vi "InitDir.vi"(8 "error in":errorcluster, 11 "DataIn":variant) -> (0 "error out":errorcluster, 3 "MainFGV_data":T1={"TestDir"=path "", "TestName"="", "Simulation"=FALSE, "task"="", "data_file"=refnum, "burts_file"=refnum, "log_file"=refnum, "Rate"=0.0, "SamplesPerChannel"=0.0, "AcqQueue"=refnum, "StartTime"=timestamp(0 s since 1904-01-01), "config_channels"=[], "DAQmx Device"="", "delta_burst"=15.0})   [LabVIEW 2016]
uses:
  MainFGV_data.ctl
  Settings/config_board.ctl
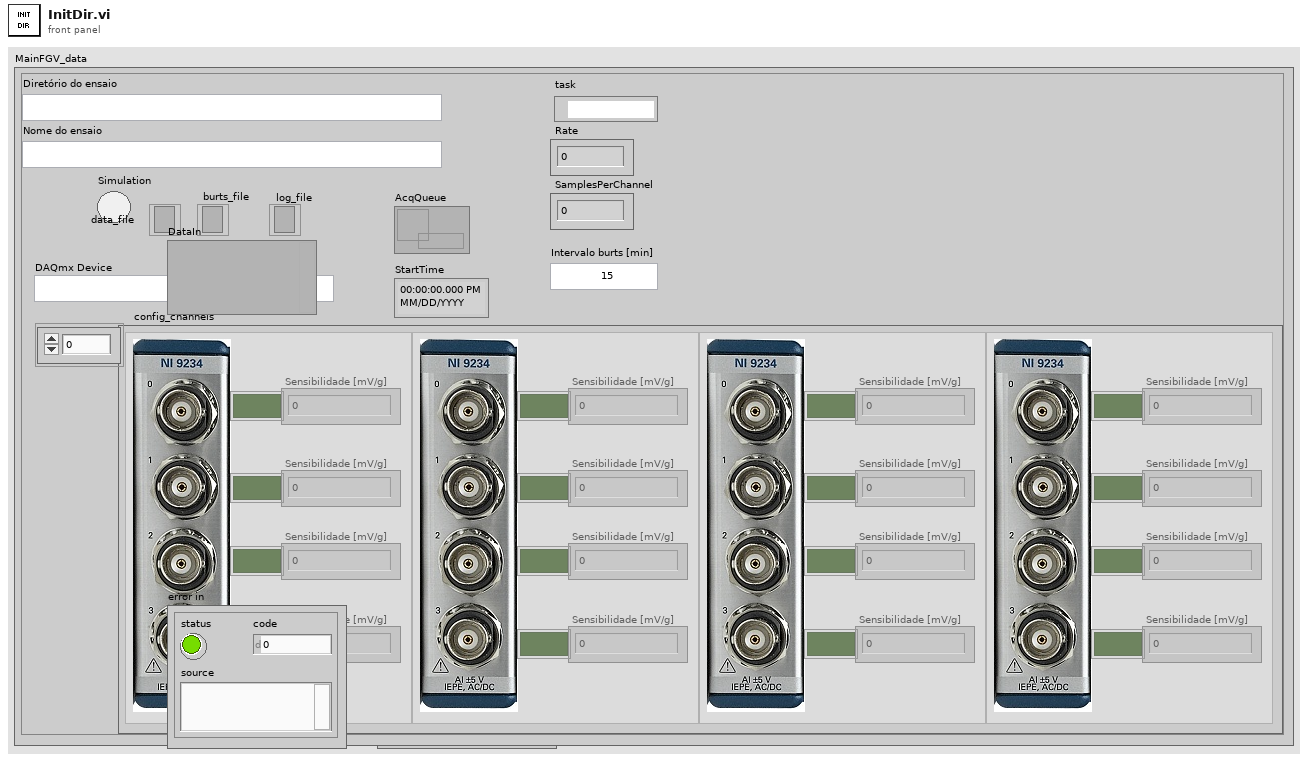
[diagram p1: front panel]
types:
  T1 = typedef "MainFGV_data.ctl" = cluster{"TestDir":path, "TestName":string, "Simulation":bool, "task":refnum<k21>, "data_file":refnum<file>, "burts_file":refnum<file>, "log_file":refnum<file>, "Rate":dbl, "SamplesPerChannel":dbl, "AcqQueue":refnum<queue>, "StartTime":timestamp, "config_channels":T2[], "DAQmx Device":tag, "delta_burst":dbl}
  T2 = typedef "config_board.ctl" = cluster{"Sens0":dbl, "Active0":bool, "Sens1":dbl, "Active1":bool, "Sens2":dbl, "Active2":bool, "Sens3":dbl, "Active3":bool}
  T3 = cluster{"simulation":bool, "TesrtDir":path, "TestName":string}
  T4 = enum16{"open", "replace", "create", "open or create", "replace or create", "replace or create with confirmation"}
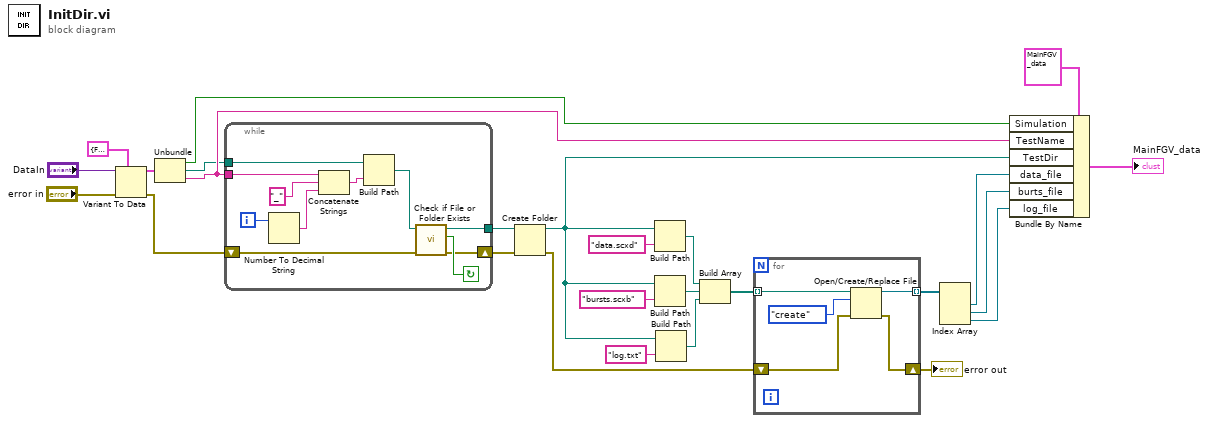
[diagram p0: block diagram]
diagram:
  n1 = Variant To Data(error in="error in", type=T3 {"simulation"=FALSE, "TesrtDir"=path "", "TestName"=""} ("output cluster"), Variant="DataIn") -> (data=w18:T3, error out=w20:errorcluster)
  n2 = Unbundle(w18) -> ("simulation"=w24:bool, "TesrtDir"=w22:path, "TestName"=w23:string)
  n3 = while {
    tunnel: w23 -> [w36]
    tunnel: w22 -> [w34]
    shift-right: [w30] -> w26
    shift-left: w20 -> [w32]
    tunnel: [w29] -> w25
    i -> [w37]
    stop <- w31 continue-if-true
    n4 = Number To Decimal String(number=w37) -> (decimal integer string=w28:string)  [unwired: 1 in]
    n5 = Concatenate Strings(w36, "_" ("string"), w28) -> (w35:string)
    n6 = Build Path(base path=w34, name or relative path=w35) -> (appended path=w33:path)
    n7 = call <vilib>:"Check if File or Folder Exists.vi"("error in (no error)"=w32, "path"=w33) -> ("error out"=w30:errorcluster, "file or folder exists?"=w31:bool, "dup path"=w29:path)  [unwired: 7 in]
  }
  n8 = Create Folder(path (use dialog)=w25, error in=w26) -> (created path=w11:path, error out=w6:errorcluster)  [unwired: 1 in, 1 out]
  n9 = Build Path(base path=w11, name or relative path="data.scxd") -> (appended path=w9:path)
  n10 = Build Path(base path=w11, name or relative path="bursts.scxb") -> (appended path=w10:path)
  n11 = Build Path(base path=w11, name or relative path="log.txt") -> (appended path=w8:path)
  n12 = Build Array(w9, w10, w8) -> (w7:path[])
  n13 = for {
    tunnel: w7 -> [w41] mode=indexing
    shift-right: [w39] -> w4
    shift-left: w6 -> [w40]
    tunnel: [w38] -> w5 mode=indexing
    n14 = Open/Create/Replace File(file path (use dialog)=w41, error in=w40, operation (0:open)=T4."create") -> (refnum out=w38:refnum<file>, error out=w39:errorcluster)  [unwired: 3 in, 1 out]
  }
  "error out" <- w4
  n15 = Index Array(array=w5) -> (element #1=w3:refnum<file>, element #2=w2:refnum<file>, element #3=w1:refnum<file>)  [unwired: 3 in]
  n16 = Bundle By Name(cluster=T1 {"TestDir"=path "", "TestName"="", "Simulation"=FALSE, "task"="", "data_file"=refnum, "burts_file"=refnum, "log_file"=refnum, "Rate"=0.0, "SamplesPerChannel"=0.0, "AcqQueue"=refnum, "StartTime"=timestamp(0 s since 1904-01-01), "config_channels"=[], "DAQmx Device"="", "delta_burst"=15.0} ("MainFGV_data"), "Simulation"=w24, "TestName"=w23, "TestDir"=w11, "data_file"=w3, "burts_file"=w2, "log_file"=w1) -> (→"MainFGV_data":T1)
